vi "Adapt To Type.vi"(7 "Type and Defaults":variant, 8 "error in (no error)":errorcluster, 10 "Variant in":variant, 11 "Deserializer in":refnum<class "JSON Deserializer.lvclass">) -> (0 "error out":errorcluster, 2 "Variant out":variant, 3 "Deserializer out":refnum<class "JSON Deserializer.lvclass">)   [LabVIEW 2019, in "JKI JSON Serialization.lvlib" / "JSON Deserializer.lvclass"]
doc: "Adapts <b>Variant in</b> previously unflattened from a JSON formatted string to match the type of <b>Type and Defaults</b>. For any cluster element in Type and Defaults, the value of the element in Type and Default is used if element with the same name is not present in Variant in. \n\nJKI JSON 1.1.10.37\nTomi Maila - JKI\nCopyright (c) 2017, JKI"
uses:
  JSON Deserializer.lvclass
  JSON Deserializer.lvclass/JSON Deserializer.ctl
  Library/Waveform Cluster.ctl
  Library/Empty Cluster.vi
  Library/Null Value.vi
  <vilib>/Utility/VariantDataType/VariantType.lvlib
  JKI JSON Serialization.lvlib
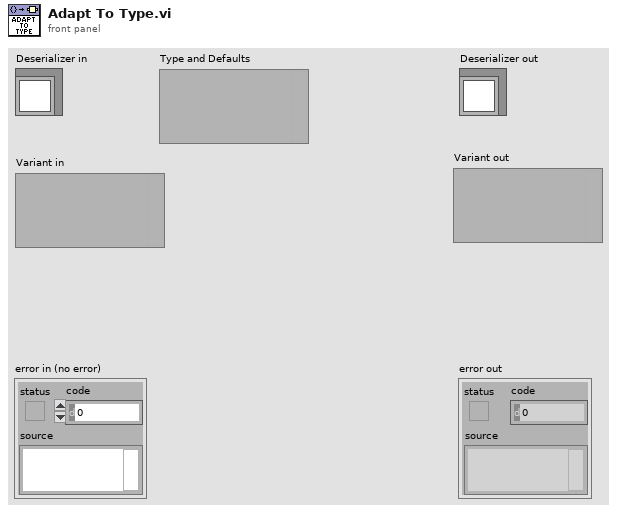
[diagram p1: front panel]
types:
  T1 = typedef "VariantType.lvlib/Type.ctl" = enum8{"Invalid Type", "Void", "I8", "I16", "I32", "I64", "U8", "U16", "U32", "U64", "Single Float", "Double Float", "Extended Float", "Single Complex", "Double Complex", "Extended Complex", "Enum U8", "Enum U16", "Enum U32", "Enum U64", "Single Float With Unit", "Double Float With Unit", "Extended Float With Unit", "Single Complex with Unit", "Double Complex with Unit", "Extended Complex with Unit", "Boolean", "String", "Path", "Picture", "Tag", "Array", "Cluster", "Variant", "LV Variant", "Waveform", "Timestamp", "Digital Waveform", "Digital Data", "ExpressData", "Refnum", "External Data", "VI", "Poly VI", "LabVIEW Class Instance", "Fixed Point"}
  T2 = typedef "JKI JSON Serialization.lvlib/Waveform Cluster.ctl" = cluster{"t0":timestamp, "dt":dbl, "y":dbl[]}
  T3 = typedef "VariantType.lvlib/MemoryInfo.ctl" = cluster{"Type":T4, "Size":u32}
  T4 = typedef "VariantType.lvlib/MemoryType.ctl" = enum16{"Variable", "Fixed", "Bounded"}
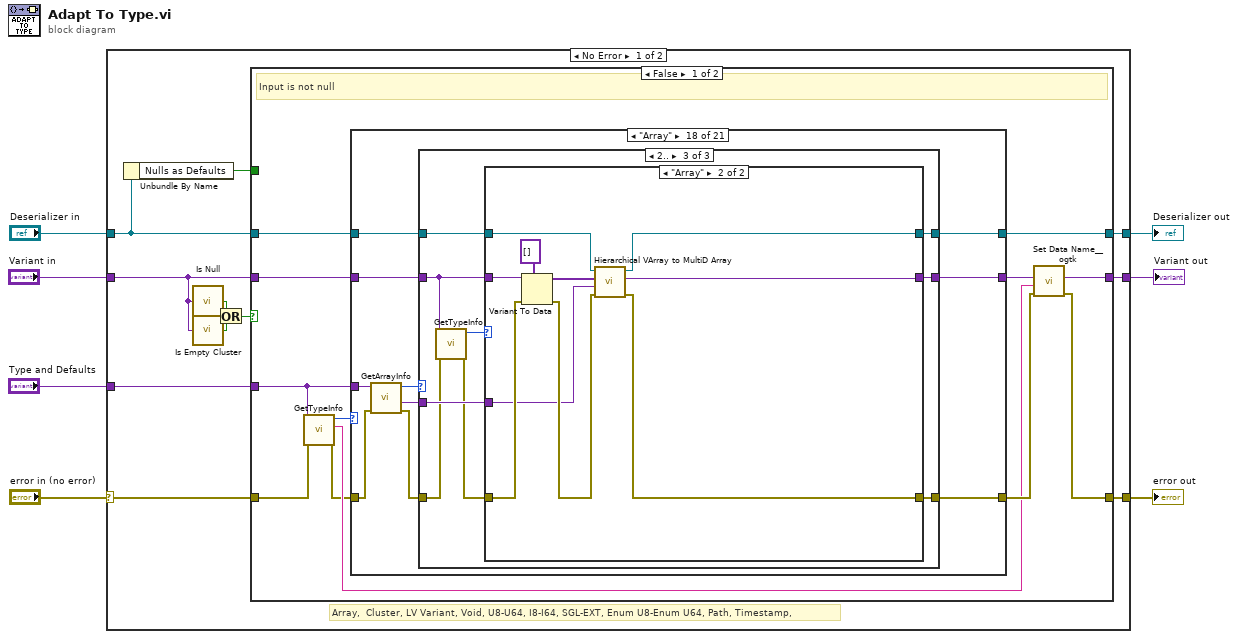
[diagram p0: block diagram]
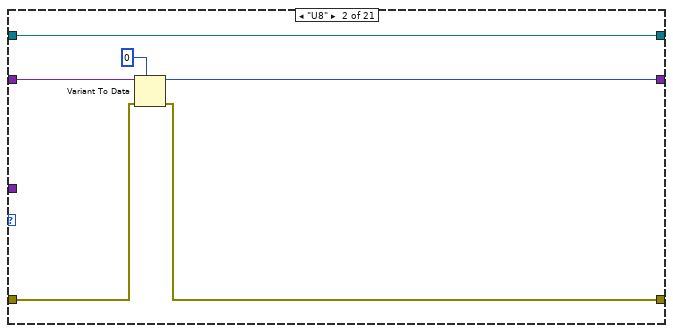
[diagram p3: hidden frame]
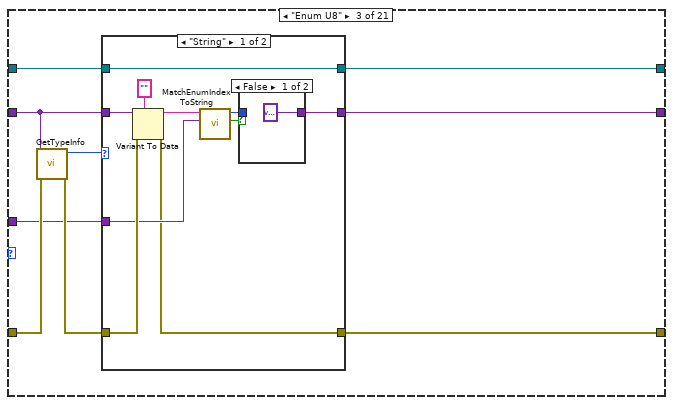
[diagram p4: hidden frame]
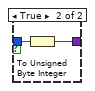
[diagram p5: hidden frame]
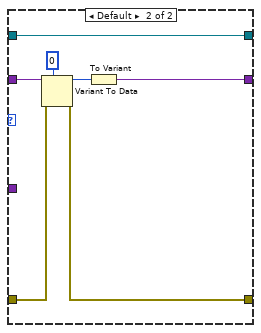
[diagram p6: hidden frame]
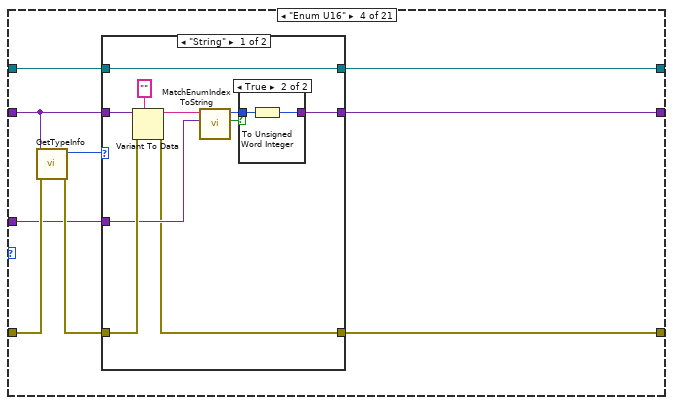
[diagram p7: hidden frame]
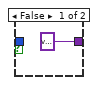
[diagram p8: hidden frame]
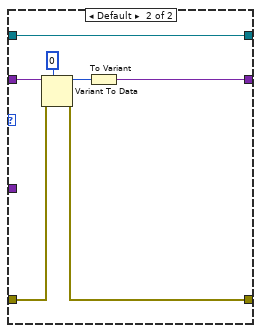
[diagram p9: hidden frame]
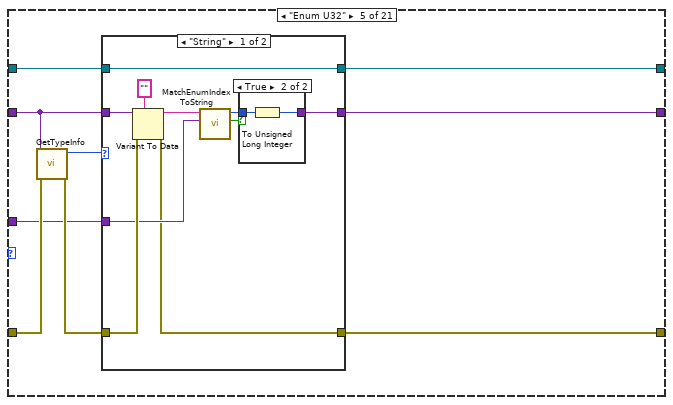
[diagram p10: hidden frame]
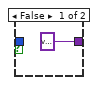
[diagram p11: hidden frame]
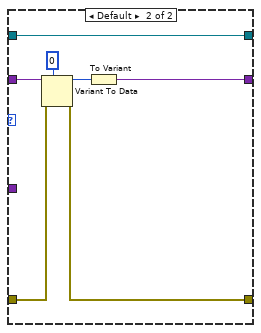
[diagram p12: hidden frame]
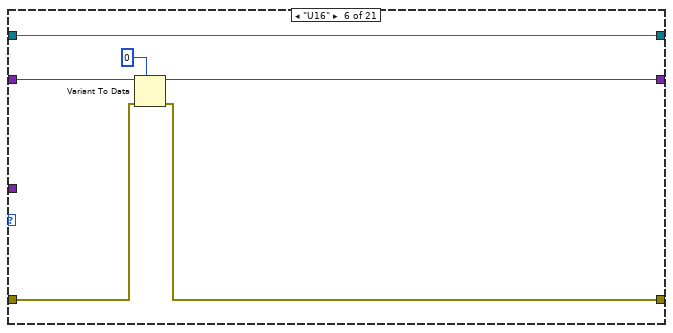
[diagram p13: hidden frame]
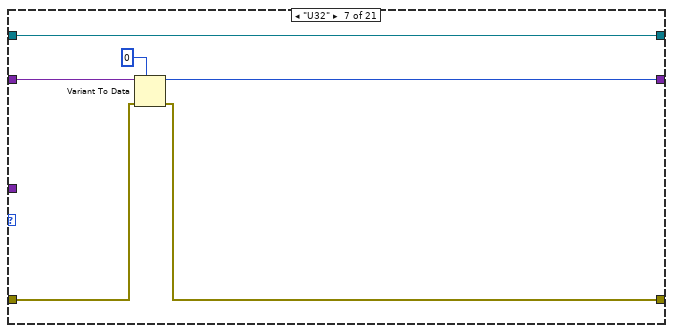
[diagram p14: hidden frame]
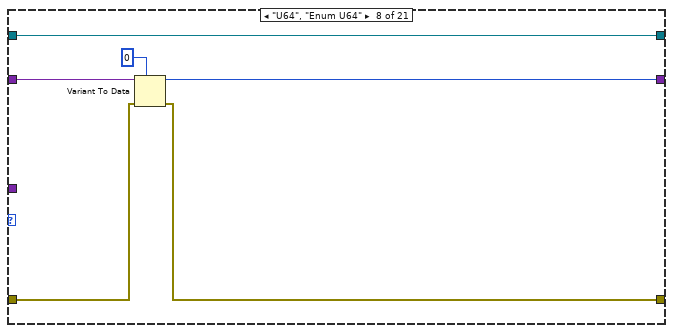
[diagram p15: hidden frame]
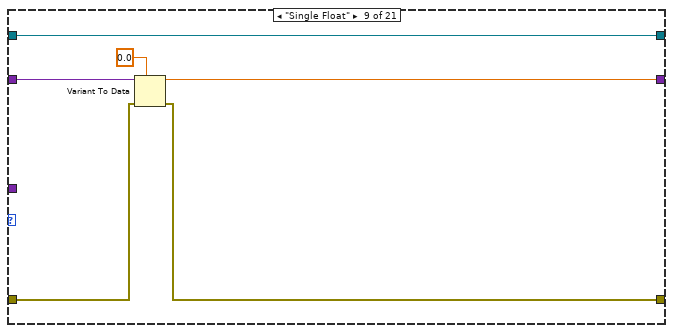
[diagram p16: hidden frame]
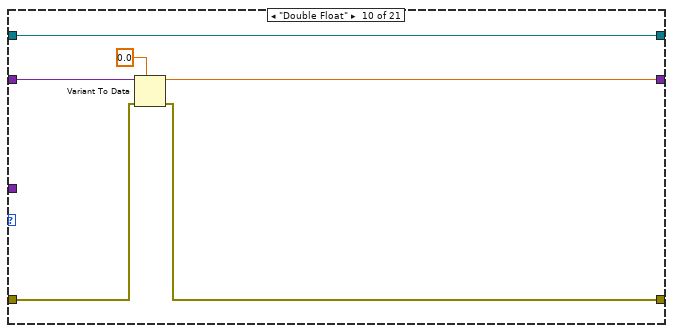
[diagram p17: hidden frame]
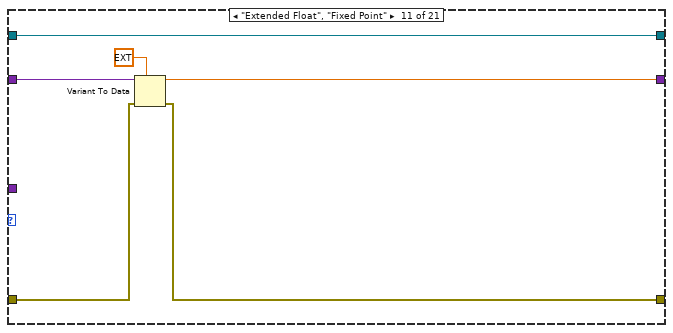
[diagram p18: hidden frame]
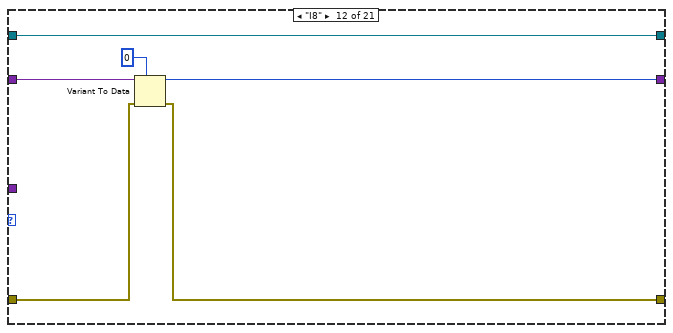
[diagram p19: hidden frame]
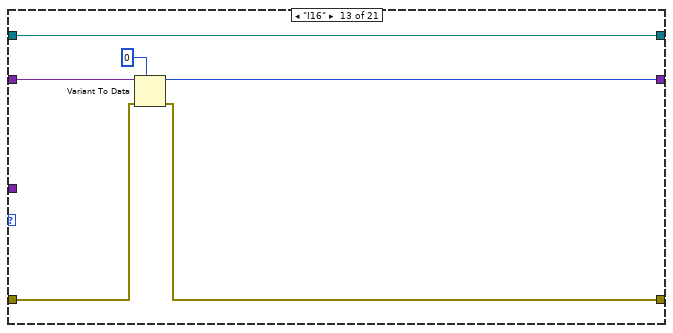
[diagram p20: hidden frame]
diagram:
  n1 = case shown="No Error" "error in (no error)" {
    selector: "error in (no error)" -> [w17 w546]
    tunnel: "Deserializer in" -> [w13 w547]
    tunnel: "Variant in" -> [w11 _]
    tunnel: [w14 w546] -> w4
    tunnel: "Type and Defaults" -> [w16 w545]
    tunnel: [w18 w547] -> w2
    tunnel: [w15 w545] -> w1
    frame No Error {
      # "Array,  Cluster, LV Variant, Void, U8-U64, I8-I64, SGL-EXT, Enum U8-Enum U64, Path, Timestamp,"
      n2 = Unbundle By Name(w13) -> ("Nulls as Defaults"=w12:bool)
      n3 = call "Is Null.vi"("Deserialized JSON Data"=w11) -> ("Null?"=w10:bool)
      n4 = call "Is Empty Cluster.vi"("Deserialized JSON Data"=w11) -> ("Empty Cluster?"=w9:bool)
      n5 = Or(x=w10, y=w9) -> (x .or. y?=w8:bool)
      n6 = case shown="False" w8 {
        tunnel: w13 -> [w20 w430]
        tunnel: [w19 w429] -> w18
        tunnel: w17 -> [w29 w427]
        tunnel: w16 -> [w28 w431]
        tunnel: [w26 w432] -> w15
        tunnel: [w25 w426] -> w14
        tunnel: w11 -> [w21 w428]
        tunnel: w12 -> [_ w425]
        frame False {
          # "Input is not null"
          n7 = call <vilib>:"GetTypeInfo.vi"("error in (no error)"=w29, "Variant"=w28) -> ("error out"=w22:errorcluster, "Name"=w23:string, "Type Enum"=w30:T1)  [unwired: 5 in, 2 out]
          n8 = case shown="\"Array\"" w30 {
            tunnel: [w32 w36 w46 w75 w104 w129 w135 w141 w147 w153 w159 w165 w171 w177 w183 w192 w195 w208 w289 w372 w422] -> w24
            tunnel: w22 -> [w32 w37 w44 w73 w102 w130 w136 w142 w148 w154 w160 w166 w172 w178 w184 w189 w199 w210 w288 w371 w422]
            tunnel: w20 -> [w33 w39 w42 w71 w100 w132 w138 w144 w150 w156 w162 w168 w174 w180 w186 w193 w201 w207 w293 w376 w424]
            tunnel: [w33 w39 w41 w70 w99 w132 w138 w144 w150 w156 w162 w168 w174 w180 w186 w193 w201 w205 w292 w375 w424] -> w19
            tunnel: w28 -> [_ _ w40 w69 w98 _ _ _ _ _ _ _ _ _ _ _ _ w211 w291 w374 _]
            tunnel: w21 -> [w31 w38 w47 w76 w105 w131 w137 w143 w149 w155 w161 w167 w173 w179 w185 w190 w200 w202 w286 w369 w423]
            tunnel: [w31 w34 w48 w77 w106 w127 w133 w139 w145 w151 w157 w163 w169 w175 w181 w191 w194 w204 w290 w373 w421] -> w27
            frame "Void", Default {
            }
            frame "U8" {
              n9 = Variant To Data(error in=w37, type=u8 0, Variant=w38) -> (data=w34:u8, error out=w36:errorcluster)
            }
            frame "Enum U8" {
              n10 = call <vilib>:"GetTypeInfo.vi"("error in (no error)"=w44, "Variant"=w47) -> ("error out"=w43:errorcluster, "Type Enum"=w45:T1)  [unwired: 5 in, 3 out]
              n11 = case shown="\"String\"" w45 {
                tunnel: [w52 w62] -> w48
                tunnel: w47 -> [w58 w66]
                tunnel: w43 -> [w56 w65]
                tunnel: [w49 w64] -> w46
                tunnel: w42 -> [w50 w63]
                tunnel: [w50 w63] -> w41
                tunnel: w40 -> [w54 _]
                frame "String" {
                  n12 = Variant To Data(error in=w56, type="", Variant=w58) -> (data=w55:string, error out=w49:errorcluster)
                  n13 = call "MatchEnumIndexToString.vi"("Enum Variant"=w54, "String"=w55) -> ("found"=w51:bool, "index"=w53:i32)  [unwired: 8 in]
                  n14 = case shown="False" w51 {
                    tunnel: w53 -> [_ w61]
                    tunnel: [variant ("Type and Defaults") w60] -> w52
                    frame False {
                    }
                    frame True {
                      n15 = To Unsigned Byte Integer(number=w61) -> (unsigned 8bit integer=w60:u8)
                    }
                  }
                }
                frame Default {
                  n16 = Variant To Data(error in=w65, type=u8 0, Variant=w66) -> (data=w67:u8, error out=w64:errorcluster)
                  n17 = To Variant(anything=w67) -> (Variant=w62:variant)
                }
              }
            }
            frame "Enum U16" {
              n18 = call <vilib>:"GetTypeInfo.vi"("error in (no error)"=w73, "Variant"=w76) -> ("error out"=w72:errorcluster, "Type Enum"=w74:T1)  [unwired: 5 in, 3 out]
              n19 = case shown="\"String\"" w74 {
                tunnel: [w81 w91] -> w77
                tunnel: w76 -> [w87 w95]
                tunnel: w72 -> [w85 w94]
                tunnel: [w78 w93] -> w75
                tunnel: w71 -> [w79 w92]
                tunnel: [w79 w92] -> w70
                tunnel: w69 -> [w83 _]
                frame "String" {
                  n20 = Variant To Data(error in=w85, type="", Variant=w87) -> (data=w84:string, error out=w78:errorcluster)
                  n21 = call "MatchEnumIndexToString.vi"("Enum Variant"=w83, "String"=w84) -> ("found"=w80:bool, "index"=w82:i32)  [unwired: 8 in]
                  n22 = case shown="True" w80 {
                    tunnel: w82 -> [_ w90]
                    tunnel: [variant ("Type and Defaults") w89] -> w81
                    frame False {
                    }
                    frame True {
                      n23 = To Unsigned Word Integer(number=w90) -> (unsigned 16bit integer=w89:u16)
                    }
                  }
                }
                frame Default {
                  n24 = Variant To Data(error in=w94, type=u16 0, Variant=w95) -> (data=w96:u16, error out=w93:errorcluster)
                  n25 = To Variant(anything=w96) -> (Variant=w91:variant)
                }
              }
            }
            frame "Enum U32" {
              n26 = call <vilib>:"GetTypeInfo.vi"("error in (no error)"=w102, "Variant"=w105) -> ("error out"=w101:errorcluster, "Type Enum"=w103:T1)  [unwired: 5 in, 3 out]
              n27 = case shown="\"String\"" w103 {
                tunnel: [w110 w120] -> w106
                tunnel: w105 -> [w116 w124]
                tunnel: w101 -> [w114 w123]
                tunnel: [w107 w122] -> w104
                tunnel: w100 -> [w108 w121]
                tunnel: [w108 w121] -> w99
                tunnel: w98 -> [w112 _]
                frame "String" {
                  n28 = Variant To Data(error in=w114, type="", Variant=w116) -> (data=w113:string, error out=w107:errorcluster)
                  n29 = call "MatchEnumIndexToString.vi"("Enum Variant"=w112, "String"=w113) -> ("found"=w109:bool, "index"=w111:i32)  [unwired: 8 in]
                  n30 = case shown="True" w109 {
                    tunnel: w111 -> [_ w119]
                    tunnel: [variant ("Type and Defaults") w118] -> w110
                    frame False {
                    }
                    frame True {
                      n31 = To Unsigned Long Integer(number=w119) -> (unsigned 32bit integer=w118:u32)
                    }
                  }
                }
                frame Default {
                  n32 = Variant To Data(error in=w123, type=u32 0, Variant=w124) -> (data=w125:u32, error out=w122:errorcluster)
                  n33 = To Variant(anything=w125) -> (Variant=w120:variant)
                }
              }
            }
            frame "U16" {
              n34 = Variant To Data(error in=w130, type=u16 0, Variant=w131) -> (data=w127:u16, error out=w129:errorcluster)
            }
            frame "U32" {
              n35 = Variant To Data(error in=w136, type=u32 0, Variant=w137) -> (data=w133:u32, error out=w135:errorcluster)
            }
            frame "U64", "Enum U64" {
              n36 = Variant To Data(error in=w142, type=u64 0, Variant=w143) -> (data=w139:u64, error out=w141:errorcluster)
            }
            frame "Single Float" {
              n37 = Variant To Data(error in=w148, type=sgl 0.0, Variant=w149) -> (data=w145:sgl, error out=w147:errorcluster)
            }
            frame "Double Float" {
              n38 = Variant To Data(error in=w154, type=0.0, Variant=w155) -> (data=w151:dbl, error out=w153:errorcluster)
            }
            frame "Extended Float", "Fixed Point" {
              n39 = Variant To Data(error in=w160, type=ext 0.0, Variant=w161) -> (data=w157:ext, error out=w159:errorcluster)
            }
            frame "I8" {
              n40 = Variant To Data(error in=w166, type=i8 0, Variant=w167) -> (data=w163:i8, error out=w165:errorcluster)
            }
            frame "I16" {
              n41 = Variant To Data(error in=w172, type=i16 0, Variant=w173) -> (data=w169:i16, error out=w171:errorcluster)
            }
            frame "I32" {
              n42 = Variant To Data(error in=w178, type=0, Variant=w179) -> (data=w175:i32, error out=w177:errorcluster)
            }
            frame "I64" {
              n43 = Variant To Data(error in=w184, type=i64 0, Variant=w185) -> (data=w181:i64, error out=w183:errorcluster)
            }
            frame "Path" {
              n44 = Variant To Data(error in=w189, type="", Variant=w190) -> (data=w187:string, error out=w192:errorcluster)
              n45 = String To Path(string=w187) -> (path=w191:path)
            }
            frame "Timestamp" {
              n46 = Variant To Data(error in=w199, type="", Variant=w200) -> (data=w197:string, error out=w196:errorcluster)
              n47 = call "ISO String To Timestamp.vi"("error in (no error)"=w196, "ISO Timestamp String"=w197) -> ("error out"=w195:errorcluster, "Time Stamp"=w194:timestamp)  [unwired: 8 in]
            }
            frame "Array" {
              n48 = call <vilib>:"GetArrayInfo.vi"("error in (no error)"=w210, "Variant"=w211) -> ("error out"=w209:errorcluster, "ArrayElement"=w206:variant, "NDims"=w203:i32)  [unwired: 6 in, 1 out]
              n49 = case shown="2.." w203 {
                tunnel: w209 -> [w214 w221 w266]
                tunnel: w202 -> [w216 w219 w264]
                tunnel: [w215 w226 w271] -> w208
                tunnel: w207 -> [w217 w225 w270]
                tunnel: w206 -> [_ w224 w269]
                tunnel: [w217 w223 w268] -> w205
                tunnel: [w216 w222 w267] -> w204
                frame 0, Default {
                  n50 = call <vilib>:"Error Cluster From Error Code.vi"("error in (no error)"=w214, "error message (\"\")"="Unflattening failed. Zero dimensional arrays not supported." ("error message (\"\")"), "error code (0)"=1) -> ("error out"=w215:errorcluster)  [unwired: 6 in]
                }
                frame 1 {
                  n51 = call <vilib>:"GetTypeInfo.vi"("error in (no error)"=w221, "Variant"=w219) -> ("error out"=w220:errorcluster, "Type Enum"=w218:T1)  [unwired: 5 in, 3 out]
                  n52 = case shown="\"Array\"" w218 {
                    tunnel: [w227 w237 w255] -> w226
                    tunnel: w225 -> [w229 w235 w254]
                    tunnel: w224 -> [w228 w234 w253]
                    tunnel: [w229 w233 w252] -> w223
                    tunnel: [w228 w232 w251] -> w222
                    tunnel: w220 -> [w227 w231 w248]
                    tunnel: w219 -> [_ w230 w250]
                    frame Default {
                    }
                    frame "Array" {
                      n53 = Variant To Data(error in=w231, type=variant[] [], Variant=w230) -> (data=w238:variant[], error out=w236:errorcluster)
                      n54 = for {
                        tunnel: w238 -> [w245] mode=indexing
                        shift-right: [w243] -> w237
                        shift-left: w236 -> [w244]
                        shift-right: [w241] -> w233
                        shift-left: w235 -> [w246]
                        tunnel: w234 -> [w242]
                        tunnel: [w240] -> w232 mode=indexing
                        n55 = call-dynamic "Adapt To Type.vi"("Type and Defaults"=w242, "error in (no error)"=w244, "Variant in"=w245, "Deserializer in"=w246) -> ("error out"=w243:errorcluster, "Variant out"=w240:variant, "Deserializer out"=w241:refnum<class "JSON Deserializer.lvclass">)  [unwired: 5 in]
                      }
                    }
                    frame "Cluster" {
                      n56 = call "Cluster to Array of VData__ogtk.vi"("error in (no error)"=w248, "Cluster"=w250) -> ("error out"=w249:errorcluster, "Array of VData"=w247:variant[])  [unwired: 8 in]
                      n57 = for {
                        tunnel: w247 -> [w261] mode=indexing
                        shift-right: [w259] -> w255
                        shift-left: w249 -> [w260]
                        shift-right: [w257] -> w252
                        shift-left: w254 -> [w262]
                        tunnel: w253 -> [w258]
                        tunnel: [w256] -> w251 mode=indexing
                        n58 = call-dynamic "Adapt To Type.vi"("Type and Defaults"=w258, "error in (no error)"=w260, "Variant in"=w261, "Deserializer in"=w262) -> ("error out"=w259:errorcluster, "Variant out"=w256:variant, "Deserializer out"=w257:refnum<class "JSON Deserializer.lvclass">)  [unwired: 5 in]
                      }
                    }
                  }
                }
                frame 2.. {
                  n59 = call <vilib>:"GetTypeInfo.vi"("error in (no error)"=w266, "Variant"=w264) -> ("error out"=w265:errorcluster, "Type Enum"=w263:T1)  [unwired: 5 in, 3 out]
                  n60 = case shown="\"Array\"" w263 {
                    tunnel: [w272 w279] -> w271
                    tunnel: w270 -> [w274 w276]
                    tunnel: w269 -> [w273 w277]
                    tunnel: [w274 w275] -> w268
                    tunnel: [w273 w278] -> w267
                    tunnel: w265 -> [w272 w283]
                    tunnel: w264 -> [_ w282]
                    frame Default {
                    }
                    frame "Array" {
                      n61 = Variant To Data(error in=w283, type=variant[] [], Variant=w282) -> (data=w281:variant[], error out=w280:errorcluster)
                      n62 = call "Hierarchical VArray to MultiD Array.vi"("error in (no error)"=w280, "Element Type"=w277, "Hierarchical Array"=w281, "Deserializer in"=w276) -> ("error out"=w279:errorcluster, "MultiD Array"=w278:variant, "Deserializer out"=w275:refnum<class "JSON Deserializer.lvclass">)  [unwired: 5 in]
                    }
                  }
                }
              }
            }
            frame "Cluster" {
              n63 = call <vilib>:"GetTypeInfo.vi"("error in (no error)"=w288, "Variant"=w286) -> ("error out"=w287:errorcluster, "Type Enum"=w285:T1)  [unwired: 5 in, 3 out]
              n64 = case shown="\"Cluster\"" w285 {
                tunnel: w293 -> [w299 w302 w308 w340]
                tunnel: [w299 w302 w307 w339] -> w292
                tunnel: w291 -> [w298 w301 w314 w338]
                tunnel: [w298 w301 w305 w330] -> w290
                tunnel: [w297 w300 w303 w327] -> w289
                tunnel: w287 -> [w296 w300 w313 w326]
                tunnel: w286 -> [_ _ w315 w325]
                frame "Invalid Type", Default {
                  n65 = call <vilib>:"Error Cluster From Error Code.vi"("error in (no error)"=w296, "error message (\"\")"="Cannot deserialize the input type into a cluster." ("error message (\"\")"), "error code (0)"=1) -> ("error out"=w297:errorcluster)  [unwired: 6 in]
                }
                frame "Void" {
                  # "Empty input object, use default values"
                }
                frame "Array" {
                  n66 = call "Cluster to Array of VData__ogtk.vi"("error in (no error)"=w313, "Cluster"=w314) -> ("error out"=w312:errorcluster, "Array of VData"=w311:variant[])  [unwired: 8 in]
                  n67 = call "Array to Array of VData__ogtk.vi"("error in (no error)"=w312, "MultiD Array"=w315) -> ("error out"=w309:errorcluster, "1D Array of Variants"=w310:variant[])  [unwired: 8 in]
                  n68 = for {
                    tunnel: w311 -> [w320] mode=indexing
                    tunnel: w310 -> [w323]
                    shift-right: [w318] -> w304
                    shift-left: w309 -> [w319]
                    shift-right: [w317] -> w307
                    shift-left: w308 -> [w324]
                    tunnel: [w316] -> w306 mode=indexing
                    i -> [w322]
                    n69 = Index Array(array=w323, index=w322) -> (element=w321:variant)
                    n70 = call-dynamic "Adapt To Type.vi"("Type and Defaults"=w320, "error in (no error)"=w319, "Variant in"=w321, "Deserializer in"=w324) -> ("error out"=w318:errorcluster, "Variant out"=w316:variant, "Deserializer out"=w317:refnum<class "JSON Deserializer.lvclass">)  [unwired: 5 in]
                  }
                  n71 = call "Array of VData to VCluster__ogtk.vi"("error in (no error)"=w304, "Array"=w306) -> ("error out"=w303:errorcluster, "VCluster"=w305:variant)  [unwired: 8 in]
                }
                frame "Cluster" {
                  n72 = call "Cluster to Array of VData__ogtk.vi"("error in (no error)"=w326, "Cluster"=w338) -> ("error out"=w336:errorcluster, "Array of VData"=w337:variant[])  [unwired: 8 in]
                  n73 = call "Cluster to Array of VData__ogtk.vi"("error in (no error)"=w336, "Cluster"=w325) -> ("error out"=w332:errorcluster, "Array of VData"=w335:variant[])  [unwired: 8 in]
                  n74 = for {
                    tunnel: w335 -> [w342] mode=indexing
                    shift-right: [w343] -> w331
                    shift-left: w332 -> [w344]
                    tunnel: [w342] -> w334 mode=indexing
                    tunnel: [w341] -> w333 mode=indexing
                    n75 = call <vilib>:"GetTypeInfo.vi"("error in (no error)"=w344, "Variant"=w342) -> ("error out"=w343:errorcluster, "Name"=w341:string)  [unwired: 5 in, 3 out]
                  }
                  n76 = for {
                    shift-right: [w354] -> w328
                    shift-left: w331 -> [w349]
                    shift-right: [w353] -> w339
                    shift-left: w340 -> [w355]
                    tunnel: w337 -> [w346] mode=indexing
                    tunnel: [w352] -> w329 mode=indexing
                    tunnel: w334 -> [w347]
                    tunnel: w333 -> [w351]
                    n77 = call <vilib>:"GetTypeInfo.vi"("error in (no error)"=w349, "Variant"=w346) -> ("error out"=w348:errorcluster, "Name"=w350:string)  [unwired: 5 in, 3 out]
                    n78 = Search 1D Array(1D array=w351, element=w350) -> (index of element=w345:i32)  [unwired: 1 in]
                    n79 = case shown="0.." w345 {
                      selector: w345 -> [_ w359]
                      tunnel: w355 -> [w358 w367]
                      tunnel: [w356 w366] -> w354
                      tunnel: [w358 w365] -> w353
                      tunnel: [w357 w364] -> w352
                      tunnel: w348 -> [w356 w363]
                      tunnel: w347 -> [_ w362]
                      tunnel: w346 -> [w357 w360]
                      frame ..-1 {
                        # "Element not found"
                      }
                      frame 0.. {
                        # "Element found"
                        n80 = Index Array(array=w362, index=w359) -> (element=w361:variant)
                        n81 = call-dynamic "Adapt To Type.vi"("Type and Defaults"=w360, "error in (no error)"=w363, "Variant in"=w361, "Deserializer in"=w367) -> ("error out"=w366:errorcluster, "Variant out"=w364:variant, "Deserializer out"=w365:refnum<class "JSON Deserializer.lvclass">)  [unwired: 5 in]
                      }
                    }
                  }
                  n82 = call "Array of VData to VCluster__ogtk.vi"("error in (no error)"=w328, "Array"=w329) -> ("error out"=w327:errorcluster, "VCluster"=w330:variant)  [unwired: 8 in]
                }
              }
            }
            frame "Waveform" {
              n83 = call <vilib>:"GetTypeInfo.vi"("error in (no error)"=w371, "Variant"=w369) -> ("error out"=w370:errorcluster, "Type Enum"=w368:T1)  [unwired: 5 in, 3 out]
              n84 = case shown="\"Array\"" w368 {
                tunnel: w376 -> [w382 w385 w400 w417]
                tunnel: [w382 w385 w387 w410] -> w375
                tunnel: w374 -> [w381 w384 w402 w419]
                tunnel: [w381 w384 w386 w409] -> w373
                tunnel: [w380 w383 w388 w411] -> w372
                tunnel: w370 -> [w379 w383 w401 w418]
                tunnel: w369 -> [_ _ w398 w416]
                frame "Invalid Type", Default {
                  n85 = call <vilib>:"Error Cluster From Error Code.vi"("error in (no error)"=w379, "error message (\"\")"="Cannot deserialize the input type into a waveform." ("error message (\"\")"), "error code (0)"=1) -> ("error out"=w380:errorcluster)  [unwired: 6 in]
                }
                frame "Void" {
                  # "Empty input object, use default values"
                }
                frame "Cluster" {
                  w394 = T2 {"t0"=timestamp(0 s since 1904-01-01), "dt"=1.0, "y"=[]}  # waveform
                  n86 = Variant To Data(error in=w401, type=waveform(dbl) {"t0"=timestamp(0 s since 1904-01-01), "dt"=1.0, "Y"=[]}, Variant=w402) -> (data=w393:waveform(dbl), error out=w397:errorcluster)
                  n87 = Unbundle By Name(w393) -> ("t0"=w405:timestamp, "dt"=w404:dbl, "Y"=w403:dbl[])
                  n88 = Bundle By Name(cluster=w394, "t0"=w405, "dt"=w404, "y"=w403) -> (w399:T2)
                  n89 = call-dynamic "Adapt To Type.vi"("Type and Defaults"=w399, "error in (no error)"=w397, "Variant in"=w398, "Deserializer in"=w400) -> ("error out"=w395:errorcluster, "Variant out"=w396:variant, "Deserializer out"=w387:refnum<class "JSON Deserializer.lvclass">)  [unwired: 5 in]
                  n90 = Variant To Data(error in=w395, type=w394, Variant=w396) -> (data=w392:T2, error out=w388:errorcluster)
                  n91 = Unbundle By Name(w392) -> ("t0"=w391:timestamp, "dt"=w390:dbl, "y"=w389:dbl[])
                  n92 = Bundle By Name(cluster=w393, "t0"=w391, "dt"=w390, "Y"=w389) -> (w386:waveform(dbl))
                }
                frame "Array" {
                  n93 = Variant To Data(error in=w418, type=waveform(dbl) {"t0"=timestamp(0 s since 1904-01-01), "dt"=1.0, "Y"=[]}, Variant=w419) -> (data=w412:waveform(dbl), error out=w415:errorcluster)
                  n94 = Unbundle By Name(w412) -> ("Y"=w408:dbl[])
                  n95 = call-dynamic "Adapt To Type.vi"("Type and Defaults"=w408, "error in (no error)"=w415, "Variant in"=w416, "Deserializer in"=w417) -> ("error out"=w413:errorcluster, "Variant out"=w414:variant, "Deserializer out"=w410:refnum<class "JSON Deserializer.lvclass">)  [unwired: 5 in]
                  n96 = Variant To Data(error in=w413, type=w408, Variant=w414) -> (data=w407:dbl[], error out=w411:errorcluster)
                  n97 = Bundle By Name(cluster=w412, "Y"=w407) -> (w409:waveform(dbl))
                }
              }
            }
            frame "LV Variant" {
              n98 = To Variant(anything=w423) -> (Variant=w421:variant)
            }
          }
          n99 = call "Set Data Name__ogtk.vi"("error in (no error)"=w24, "Data Name"=w23, "Data"=w27) -> ("error out"=w25:errorcluster, "Renamed Data"=w26:variant)  [unwired: 7 in]
        }
        frame True {
          # "Input is null"
          n100 = case shown="False" w425 {
            tunnel: [w440 w544] -> w432
            tunnel: w431 -> [w437 w544]
            tunnel: w430 -> [w444 w543]
            tunnel: [w443 w543] -> w429
            tunnel: w428 -> [w442 _]
            tunnel: w427 -> [w436 w542]
            tunnel: [w438 w542] -> w426
            frame False {
              # "Return null value if supported by type"
              n101 = call <vilib>:"GetTypeInfo.vi"("error in (no error)"=w436, "Variant"=w437) -> ("error out"=w435:errorcluster, "Name"=w433:string, "Type Enum"=w434:T1)  [unwired: 5 in, 2 out]
              n102 = case shown="\"Waveform\"" w434 {
                tunnel: [w446 w448 w451 w454 w457 w460 w463 w466 w469 w472 w475 w478 w481 w484 w487 w490 w493 w498 w502 w514] -> w439
                tunnel: w435 -> [w446 w448 w451 w454 w457 w460 w463 w466 w469 w472 w475 w478 w481 w484 w487 w490 w493 w498 w505 w516]
                tunnel: w444 -> [w447 w450 w453 w456 w459 w462 w465 w468 w471 w474 w477 w480 w483 w486 w489 w492 w495 w499 w506 w513]
                tunnel: [w447 w450 w453 w456 w459 w462 w465 w468 w471 w474 w477 w480 w483 w486 w489 w492 w495 w499 w506 w511] -> w443
                tunnel: w437 -> [_ _ _ _ _ _ _ _ _ _ _ _ _ _ _ _ _ _ w501 w517]
                tunnel: w442 -> [w445 _ _ _ _ _ _ _ _ _ _ _ _ _ _ _ _ w497 _ w508]
                tunnel: [w445 "" path "" waveform(dbl) {"t0"=timestamp(0 s since 1904-01-01), "dt"=1.0, "Y"=[]} FALSE timestamp(0 s since 1904-01-01) sgl nan nan ext nan u8 0 u16 0 u32 0 u64 0 i8 0 i16 0 0 i64 0 w496 w500 w510] -> w441
                frame "Void", Default {
                }
                frame "String" {
                }
                frame "Path" {
                }
                frame "Waveform" {
                }
                frame "Boolean" {
                }
                frame "Timestamp" {
                }
                frame "Single Float" {
                }
                frame "Double Float" {
                }
                frame "Extended Float", "Fixed Point" {
                }
                frame "U8", "Enum U8" {
                }
                frame "U16", "Enum U16" {
                }
                frame "U32", "Enum U32" {
                }
                frame "U64", "Enum U64" {
                }
                frame "I8" {
                }
                frame "I16" {
                }
                frame "I32" {
                }
                frame "I64" {
                }
                frame "LV Variant" {
                  n103 = To Variant(anything=w497) -> (Variant=w496:variant)
                }
                frame "Cluster" {
                  # "Get cluster default value"
                  n104 = call <vilib>:"GetClusterInfo.vi"("error in (no error)"=w505, "Variant"=w501) -> ("error out"=w503:errorcluster, "Cluster Elements"=w504:variant[])  [unwired: 8 in]
                  n105 = call <vilib>:"SetClusterInfo.vi"("error in (no error)"=w503, "Cluster Elements"=w504, "Variant"=w501) -> ("error out"=w502:errorcluster, "Variant Out"=w500:variant)  [unwired: 7 in]
                }
                frame "Array" {
                  n106 = call <vilib>:"GetArrayInfo.vi"("error in (no error)"=w516, "Variant"=w517) -> ("error out"=w515:errorcluster, "ArrayElement"=w512:variant, "Array Lengths"=w507:T3[], "NDims"=w509:i32)  [unwired: 6 in]
                  n107 = case shown="0, Default" w509 {
                    tunnel: w515 -> [w520 w527 w540]
                    tunnel: w508 -> [w522 _ _]
                    tunnel: [w521 w524 w534] -> w514
                    tunnel: w513 -> [w523 w528 w541]
                    tunnel: w512 -> [_ w526 w539]
                    tunnel: [w523 w528 w541] -> w511
                    tunnel: [w522 w529 w536] -> w510
                    tunnel: w507 -> [_ _ w533]
                    frame 0, Default {
                      n108 = call <vilib>:"Error Cluster From Error Code.vi"("error in (no error)"=w520, "error message (\"\")"="Unflattening failed. Zero dimensional arrays not supported." ("error message (\"\")"), "error code (0)"=1) -> ("error out"=w521:errorcluster)  [unwired: 6 in]
                    }
                    frame 1 {
                      n109 = call "Array of VData to VArray__ogtk.vi"("error in (no error)"=w527, "Element Type (when empty)"=w526, "1D Array of VData"=variant[] []) -> ("error out"=w524:errorcluster, "VArray"=w529:variant)  [unwired: 7 in]
                    }
                    frame 2.. {
                      n110 = Array Size(array=w533) -> (size(s)=w532:i32)
                      n111 = Initialize Array(0, w532) -> (w530:i32[])
                      n112 = call "Array of VData to VArray__ogtk.vi"("error in (no error)"=w540, "Element Type (when empty)"=w539, "1D Array of VData"=variant[] []) -> ("error out"=w535:errorcluster, "VArray"=w537:variant)  [unwired: 7 in]
                      n113 = call "Reshape 1D Array__ogtk.vi"("error in (no error)"=w535, "Size(s)"=w530, "1D Array"=w537) -> ("error out"=w534:errorcluster, "Reshaped VArray"=w536:variant)  [unwired: 7 in]
                    }
                  }
                }
              }
              n114 = call "Set Data Name__ogtk.vi"("error in (no error)"=w439, "Data Name"=w433, "Data"=w441) -> ("error out"=w438:errorcluster, "Renamed Data"=w440:variant)  [unwired: 7 in]
            }
            frame True {
              # "Return default value"
            }
          }
        }
      }
    }
    frame Error {
    }
  }
  "error out" <- w4
  "Deserializer out" <- w2
  "Variant out" <- w1
